vi "TableStrAdd.vi"(2 "error in":errorcluster caption="错误输入（无错误）", 3 "Array":string[][](array[string])) -> (0 "error out":errorcluster caption="错误输出", 1 "数组":string[][](array[string]))   [LabVIEW 2013]
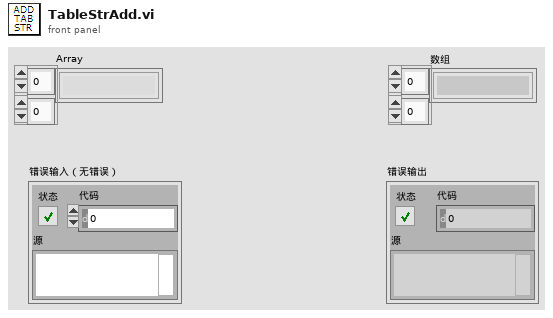
[diagram p1: front panel]
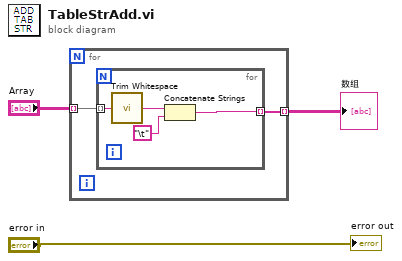
[diagram p0: block diagram]
diagram:
  n1 = for {
    tunnel: "Array" -> [w5] mode=indexing
    tunnel: [w4] -> w2 mode=indexing
    n2 = for {
      tunnel: w5 -> [w9] mode=indexing
      tunnel: [w8] -> w4 mode=indexing
      n3 = call <vilib>:"Trim Whitespace.vi"("string"=w9) -> ("trimmed string"=w7:string)  [unwired: 1 in]
      n4 = Concatenate Strings(w7, "\t") -> (w8:string)
    }
  }
  "数组" <- w2
  "error out" <- "error in"
